vi "Autonomous Independent.vi"   [LabVIEW 2011]
doc: "This VI is called when autonomous begins, and will automatically be terminated when autonomous ends. You can carry out timed or sensor driven robot movement independently without needing to return to the caller."
uses:
  Robot Global Data.vi
  System Set Points and States.vi
types:
  T1 = typedef "WPI_DigitalInputDevRef.ctl" = cluster{"DevStatus":errorcluster, "DIO Channel":T2, "Digital Module":T3}
  T2 = typedef "FPGA_DIOChannel.ctl" = enum8{"DIO 1", "DIO 2", "DIO 3", "DIO 4", "DIO 5", "DIO 6", "DIO 7", "DIO 8", "DIO 9", "DIO 10", "DIO 11", "DIO 12", "DIO 13", "DIO 14", "Invalid"}
  T3 = typedef "FPGA_TypedefDigitalModule.ctl" = enum16{"Digital Module 1", "Digital Module 2"}
  T4 = typedef "WPI_MotorControlDeviceRef.ctl" = cluster{"DeviceStatus":errorcluster, "Type":enum16{"PWM", "CAN"}, "PWM":cluster{"Digital Module":T3, "PWM Channel":T5, "DeadBand":T6}, "CAN":cluster{"Device Number":u8, "Control Mode":T7, "Semaphore":T8, "Max Vout":dbl}, "Invert":bool, "TransformRef":T9, "InvTransformRef":T9}
  T5 = typedef "FPGA_DIOPWMChannel.ctl" = enum8{"PWM 1", "PWM 2", "PWM 3", "PWM 4", "PWM 5", "PWM 6", "PWM 7", "PWM 8", "PWM 9", "PWM 10", "Invalid"}
  T6 = typedef "WPI_PWMDeadband.ctl" = cluster{"Name":string, "maxPositivePwm":i32, "minPositivePwm":i32, "centerPwm":i32, "maxNegativePwm":i32, "minNegativePwm":i32, "angularRange":u16}
  T7 = typedef "WPI_CANJaguar_ControlMode.ctl" = enum8{"Percent VBus", "Current", "Speed", "Position", "Voltage"}
  T8 = typedef "Semaphore RefNum" = refnum<k1>
  T9 = typedef "WPI_PWMTransform_ConPane.ctl" = refnum<vi>
  T10 = typedef "WPI_AnalogChannelDevRef.ctl" = cluster{"DevStatus":errorcluster, "Analog Module":T11, "Analog Channel":T12}
  T11 = typedef "FPGA_TypedefAnalogModule.ctl" = enum16{"Analog Module 1", "Analog Module 2"}
  T12 = typedef "FPGA_AIChannel.ctl" = enum8{"AI 1", "AI 2", "AI 3", "AI 4", "AI 5", "AI 6", "AI 7", "AI 8", "Invalid"}
  T13 = typedef "WPI_RobotDriveDevRef.ctl" = cluster{"DevStatus":errorcluster, "Motors[]":T4[], "Square Inputs":bool, "Max Output":dbl, "Isochronous":bool}
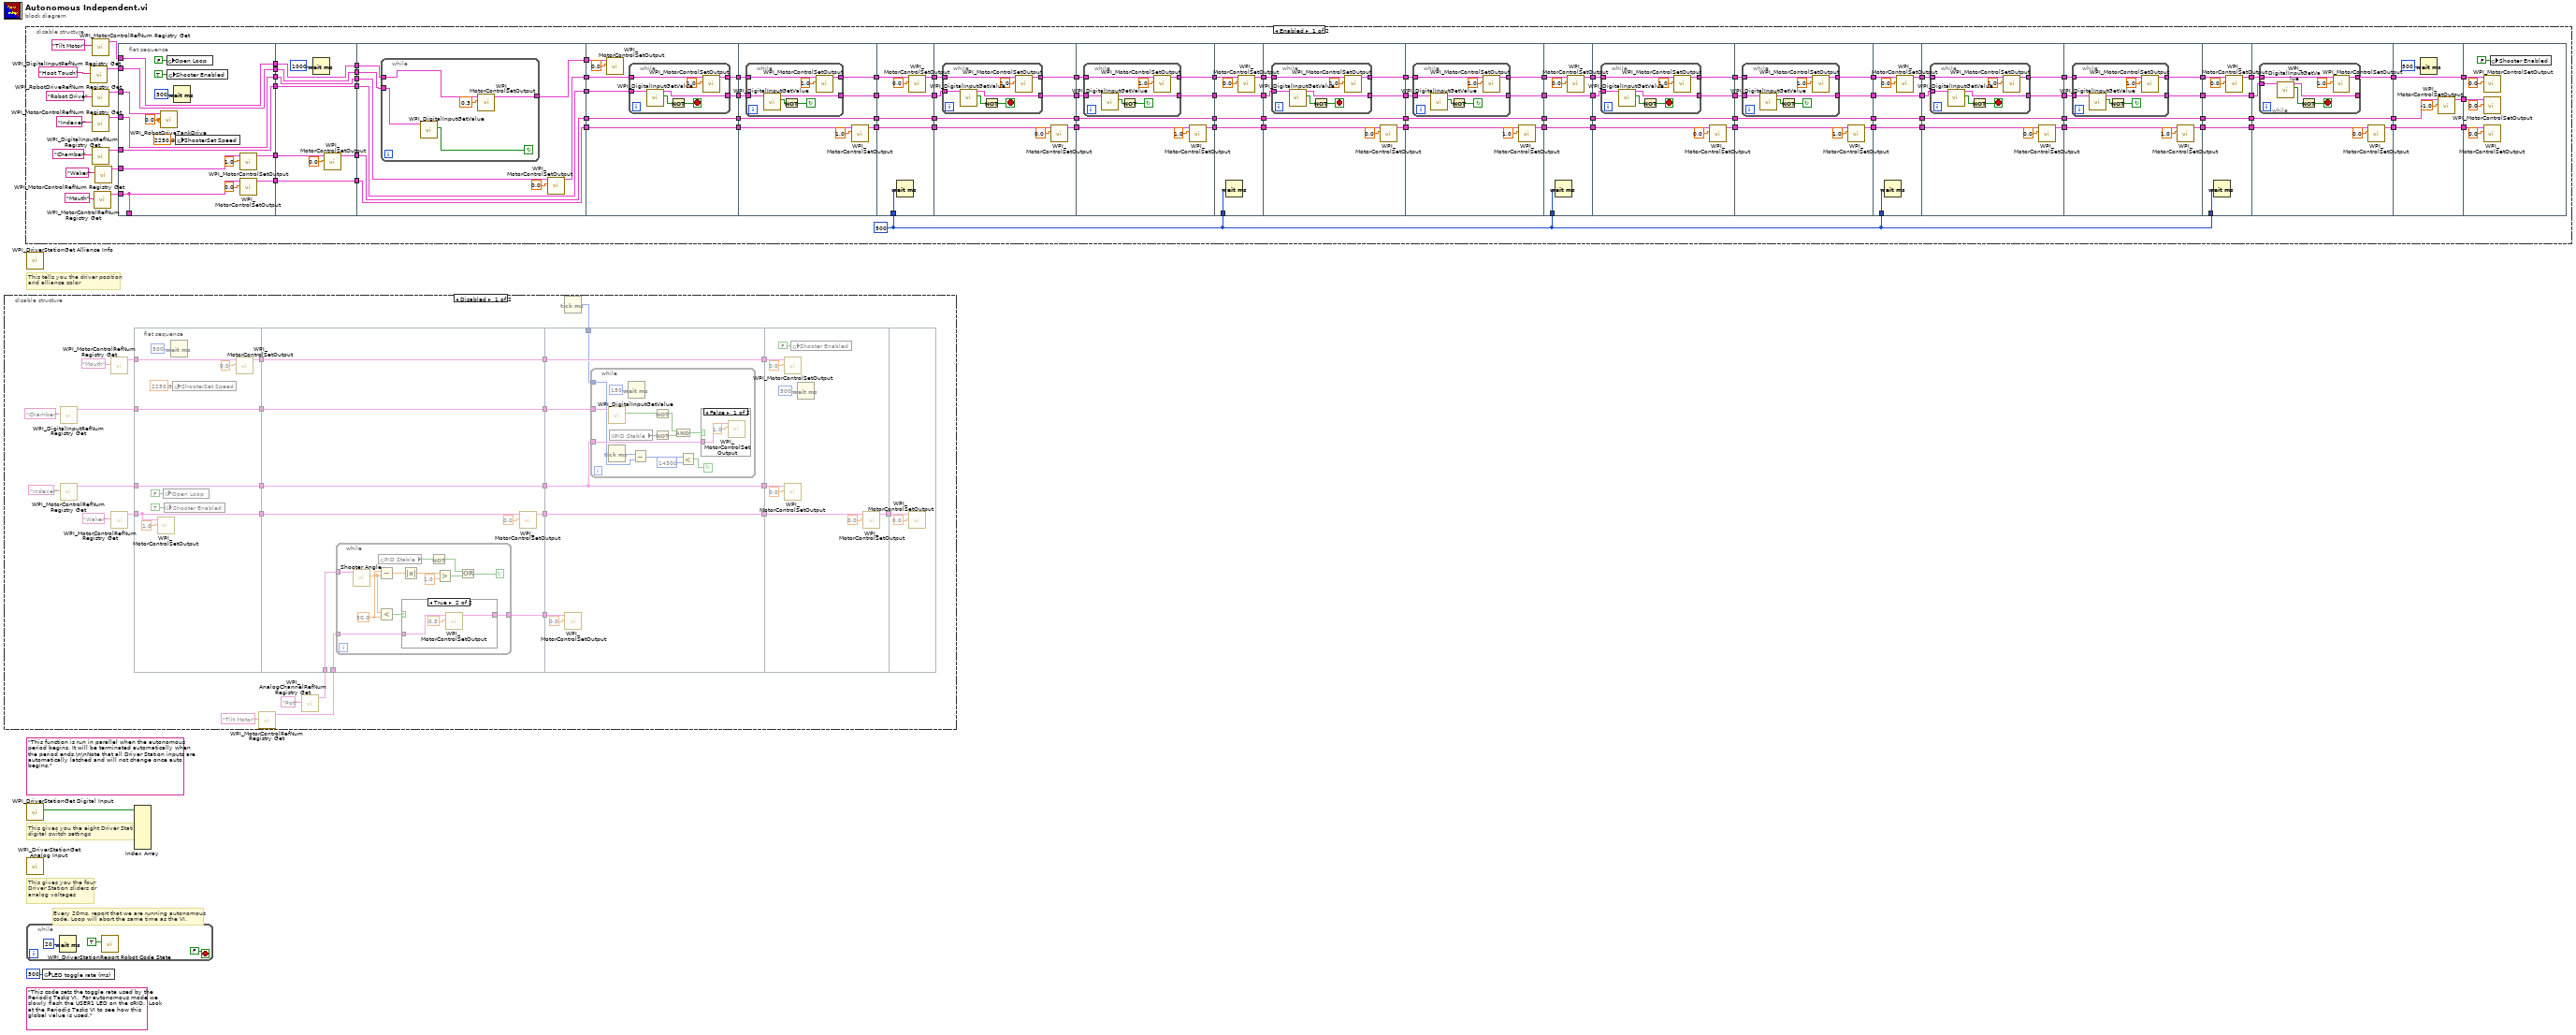
[diagram p0: block diagram]
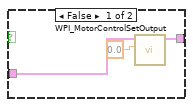
[diagram p2: hidden frame]
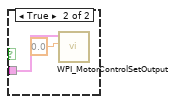
[diagram p3: hidden frame]
diagram:
  (unwired) "This function is run in parallel when the autonomous period begins. It will be terminated automatically when the period ends.\n\nNote that all Driver Station inputs are automatically latched and will not change once auto begins."
  (unwired) "This code sets the toggle rate used by the Periodic Tasks VI.  For autonomous mode we slowly flash the USER1 LED on the cRIO.  Look at the Periodic Tasks VI to see how this global value is used."
  # "Every 20ms, report that we are running autonomous\ncode. Loop will abort the same time as the VI."
  # "This tells you the driver position\nand alliance color"
  # "This gives you the eight Driver Station\ndigital switch settings"
  # "This gives you the four\nDriver Station sliders or\nanalog voltages"
  n1 = disable-structure shown="Disabled" {
    frame Disabled {
      n2 = call <vilib>:"WPI_DigitalInputRefNum Registry Get.vi"("refnum name"="Chamber") -> ("DigitalInputDevRef"=w12:T1)  [unwired: 9 in, 1 out]
      n3 = call <vilib>:"WPI_MotorControlRefNum Registry Get.vi"("refnum name"="Indexer") -> ("MotorControlDevRef"=w9:T4)  [unwired: 9 in, 1 out]
      n4 = call <vilib>:"WPI_MotorControlRefNum Registry Get.vi"("refnum name"="Mouth") -> ("MotorControlDevRef"=w7:T4)  [unwired: 9 in, 1 out]
      n5 = call <vilib>:"WPI_MotorControlRefNum Registry Get.vi"("refnum name"="Waker") -> ("MotorControlDevRef"=w8:T4)  [unwired: 9 in, 1 out]
      n6 = flat-sequence {
        tunnel: w9 -> [w34]
        tunnel: w8 -> [w32]
        tunnel: w12 -> [w33]
        tunnel: [w34] -> w28
        tunnel: [w33] -> w27
        tunnel: [w32] -> w26
        tunnel: w7 -> [w30]
        tunnel: [w29] -> w25
        tunnel: w28 -> [w48]
        tunnel: [w48] -> w24
        tunnel: w27 -> [w47]
        tunnel: [w47] -> w23
        tunnel: w26 -> [w46]
        tunnel: [w44] -> w22
        tunnel: w25 -> [w44]
        tunnel: w5 -> [w43]
        tunnel: w3 -> [w42]
        tunnel: [w41] -> w21
        tunnel: [w40] -> w20
        tunnel: w24 -> [w73]
        tunnel: w23 -> [w74]
        tunnel: [w73] -> w19
        tunnel: [w72] -> w18
        tunnel: w22 -> [w72]
        tunnel: w10 -> [w71]
        tunnel: w21 -> [w69]
        tunnel: [w68] -> w17
        tunnel: w20 -> [w68]
        tunnel: w19 -> [w98]
        tunnel: w18 -> [w96]
        tunnel: w17 -> [w93]
        tunnel: [w92] -> w16
        tunnel: w16 -> [w102]
        frame #0 {
          n7 = call <vilib>:"WPI_MotorControlSetOutput.vi"("Output"=1.0, "MotorControlDevRef"=w32) -> ()  [unwired: 8 in, 2 out]
          n8 = global write "System Set Points and States.vi" "Open Loop"(FALSE ("Open Loop")) -> ()
          n9 = global write "System Set Points and States.vi" "Shooter Enabled"(TRUE ("Shooter Enabled")) -> ()
          n10 = Wait (ms)(milliseconds to wait=u32 500) -> ()  [unwired: 1 out]
          n11 = global write "System Set Points and States.vi" "ShooterSet Speed"(2250.0) -> ()
          n12 = call <vilib>:"WPI_MotorControlSetOutput.vi"("Output"=0.0, "MotorControlDevRef"=w30) -> ("MotorControlDevRef"=w29:T4)  [unwired: 8 in, 1 out]
        }
        frame #1 {
          n13 = while {
            tunnel: w43 -> [w56]
            tunnel: w42 -> [w55]
            tunnel: [w54] -> w41
            stop <- w49 continue-if-true
            w58 = 50.0 ("y")
            n14 = call "Shooter Angle.vi"("AIDeviceRef"=w56) -> ("Shoter Angle"=w57:dbl)  [unwired: 9 in, 1 out]
            n15 = Subtract(x=w58, y=w57) -> (x-y=w59:dbl)
            n16 = Less?(x=w57, y=w58) -> (x < y?=w60:bool)
            n17 = global read "System Set Points and States.vi" "PID Stable"() -> (w61:bool)
            n18 = case shown="True" w60 {
              tunnel: w55 -> [w63 w66]
              tunnel: [w62 w65] -> w54
              frame False {
                n19 = call <vilib>:"WPI_MotorControlSetOutput.vi"("Output"=0.0, "MotorControlDevRef"=w63) -> ("MotorControlDevRef"=w62:T4)  [unwired: 8 in, 1 out]
              }
              frame True {
                n20 = call <vilib>:"WPI_MotorControlSetOutput.vi"("Output"=0.3, "MotorControlDevRef"=w66) -> ("MotorControlDevRef"=w65:T4)  [unwired: 8 in, 1 out]
              }
            }
            n21 = Absolute Value(x=w59) -> (abs(x)=w53:dbl)
            n22 = Not(x=w61) -> (.not. x?=w50:bool)
            n23 = Greater?(x=w53, y=1.0) -> (0:w51:bool)
            n24 = Or(x=w50, y=w51) -> (x .or. y?=w49:bool)
          }
          n25 = call <vilib>:"WPI_MotorControlSetOutput.vi"("Output"=0.0, "MotorControlDevRef"=w46) -> ("MotorControlDevRef"=w40:T4)  [unwired: 8 in, 1 out]
        }
        frame #2 {
          n26 = call <vilib>:"WPI_MotorControlSetOutput.vi"("Output"=0.0, "MotorControlDevRef"=w69) -> ()  [unwired: 8 in, 2 out]
          n27 = while {
            tunnel: w74 -> [w87]
            tunnel: w73 -> [w86]
            tunnel: w71 -> [w77]
            stop <- w84 continue-if-true
            n28 = call <vilib>:"WPI_DigitalInputGetValue.vi"("DigitalInputDevRef"=w87) -> ("Value"=w83:bool)  [unwired: 8 in, 2 out]
            n29 = Tick Count (ms)() -> (millisecond timer value=w76:u32)
            n30 = global read "System Set Points and States.vi" "PID Stable"() -> (w81:bool)
            n31 = Wait (ms)(milliseconds to wait=u32 150) -> ()  [unwired: 1 out]
            n32 = Subtract(x=w76, y=w77) -> (x-y=w78:u32)
            n33 = Not(x=w83) -> (.not. x?=w82:bool)
            n34 = Not(x=w81) -> (.not. x?=w80:bool)
            n35 = And(x=w82, y=w80) -> (x .and. y?=w79:bool)
            n36 = Less?(x=w78, y=u32 14300) -> (x < y?=w84:bool)
            n37 = case shown="False" w79 {
              tunnel: w86 -> [w89 w91]
              frame False {
                n38 = call <vilib>:"WPI_MotorControlSetOutput.vi"("Output"=1.0, "MotorControlDevRef"=w89) -> ()  [unwired: 8 in, 2 out]
              }
              frame True {
                n39 = call <vilib>:"WPI_MotorControlSetOutput.vi"("Output"=0.0, "MotorControlDevRef"=w91) -> ()  [unwired: 8 in, 2 out]
              }
            }
          }
        }
        frame #3 {
          n40 = call <vilib>:"WPI_MotorControlSetOutput.vi"("Output"=0.0, "MotorControlDevRef"=w96) -> ()  [unwired: 8 in, 2 out]
          n41 = call <vilib>:"WPI_MotorControlSetOutput.vi"("Output"=0.0, "MotorControlDevRef"=w98) -> ()  [unwired: 8 in, 2 out]
          n42 = global write "System Set Points and States.vi" "Shooter Enabled"(FALSE ("Shooter Enabled")) -> ()
          n43 = Wait (ms)(milliseconds to wait=u32 500) -> ()  [unwired: 1 out]
          n44 = call <vilib>:"WPI_MotorControlSetOutput.vi"("Output"=0.0, "MotorControlDevRef"=w93) -> ("MotorControlDevRef"=w92:T4)  [unwired: 8 in, 1 out]
        }
        frame #4 {
          n45 = call <vilib>:"WPI_MotorControlSetOutput.vi"("Output"=0.0, "MotorControlDevRef"=w102) -> ()  [unwired: 8 in, 2 out]
        }
      }
      n46 = call <vilib>:"WPI_MotorControlRefNum Registry Get.vi"("refnum name"="Tilt Motor") -> ("MotorControlDevRef"=w3:T4)  [unwired: 9 in, 1 out]
      n47 = call <vilib>:"WPI_AnalogChannelRefNum Registry Get.vi"("refnum name"="Pot") -> ("AIDeviceRef"=w5:T10)  [unwired: 9 in, 1 out]
      n48 = Tick Count (ms)() -> (millisecond timer value=w10:u32)
    }
    frame Enabled {
    }
  }
  n49 = disable-structure shown="Enabled" {
    frame Enabled {
      w107 = u32 500 ("milliseconds to wait")
      n50 = call <vilib>:"WPI_DigitalInputRefNum Registry Get.vi"("refnum name"="Hoot Touch") -> ("DigitalInputDevRef"=w103:T1)  [unwired: 9 in, 1 out]
      n51 = call <vilib>:"WPI_MotorControlRefNum Registry Get.vi"("refnum name"="Tilt Motor") -> ("MotorControlDevRef"=w113:T4)  [unwired: 9 in, 1 out]
      n52 = call <vilib>:"WPI_RobotDriveRefNum Registry Get.vi"("refnum name"="Robot Drive") -> ("RobotDriveDevRef"=w108:T13)  [unwired: 9 in, 1 out]
      n53 = call <vilib>:"WPI_MotorControlRefNum Registry Get.vi"("refnum name"="Indexer") -> ("MotorControlDevRef"=w112:T4)  [unwired: 9 in, 1 out]
      n54 = call <vilib>:"WPI_DigitalInputRefNum Registry Get.vi"("refnum name"="Chamber") -> ("DigitalInputDevRef"=w116:T1)  [unwired: 9 in, 1 out]
      n55 = call <vilib>:"WPI_MotorControlRefNum Registry Get.vi"("refnum name"="Mouth") -> ("MotorControlDevRef"=w110:T4)  [unwired: 9 in, 1 out]
      n56 = call <vilib>:"WPI_MotorControlRefNum Registry Get.vi"("refnum name"="Waker") -> ("MotorControlDevRef"=w111:T4)  [unwired: 9 in, 1 out]
      n57 = flat-sequence {
        tunnel: w112 -> [w211]
        tunnel: w111 -> [w209]
        tunnel: w116 -> [w210]
        tunnel: [w211] -> w200
        tunnel: [w210] -> w199
        tunnel: [w202] -> w198
        tunnel: [w205] -> _
        tunnel: [w207] -> w197
        tunnel: [w206] -> w196
        tunnel: w113 -> [w206]
        tunnel: w110 -> [w205]
        tunnel: w108 -> [w204]
        tunnel: [w201] -> w104
        tunnel: w103 -> [w201]
        tunnel: w200 -> [w225]
        tunnel: [w225] -> w195
        tunnel: w199 -> [w224]
        tunnel: [w224] -> w194
        tunnel: w198 -> [w220]
        tunnel: w197 -> [w223]
        tunnel: [w223] -> w193
        tunnel: w196 -> [w222]
        tunnel: [w222] -> w192
        tunnel: [w219] -> w191
        tunnel: [w217] -> w105
        tunnel: w104 -> [w217]
        tunnel: w195 -> [w230]
        tunnel: [w228] -> w190
        tunnel: w194 -> [w234]
        tunnel: [w234] -> w189
        tunnel: [w233] -> w188
        tunnel: w193 -> [w233]
        tunnel: w192 -> [w232]
        tunnel: [w231] -> w187
        tunnel: [w227] -> w186
        tunnel: w191 -> [w227]
        tunnel: w105 -> [w226]
        tunnel: w190 -> [w247]
        tunnel: w189 -> [w242]
        tunnel: [w244] -> w185
        tunnel: [w243] -> w184
        tunnel: w188 -> [w243]
        tunnel: w187 -> [w245]
        tunnel: [w241] -> w183
        tunnel: [w240] -> w182
        tunnel: w186 -> [w240]
        tunnel: w185 -> [w262]
        tunnel: w184 -> [w257]
        tunnel: w183 -> [w261]
        tunnel: [w260] -> w181
        tunnel: [w259] -> w180
        tunnel: [w256] -> w179
        tunnel: [w255] -> w178
        tunnel: w182 -> [w255]
        tunnel: [w271] -> w177
        tunnel: w181 -> [w273]
        tunnel: w180 -> [w275]
        tunnel: w179 -> [w271]
        tunnel: [w274] -> w176
        tunnel: [w273] -> w175
        tunnel: w107 -> [w272]
        tunnel: [w270] -> w174
        tunnel: w178 -> [w270]
        tunnel: w177 -> [w279]
        tunnel: [w278] -> w173
        tunnel: w176 -> [w284]
        tunnel: [w283] -> w172
        tunnel: [w282] -> w171
        tunnel: w175 -> [w281]
        tunnel: [w277] -> w170
        tunnel: w174 -> [w277]
        tunnel: w173 -> [w298]
        tunnel: w172 -> [w297]
        tunnel: w171 -> [w296]
        tunnel: [w295] -> w169
        tunnel: [w294] -> w168
        tunnel: [w293] -> w167
        tunnel: [w292] -> w166
        tunnel: w170 -> [w292]
        tunnel: w169 -> [w312]
        tunnel: [w311] -> w165
        tunnel: w168 -> [w311]
        tunnel: [w310] -> w164
        tunnel: w167 -> [w308]
        tunnel: [w308] -> w163
        tunnel: w107 -> [w309]
        tunnel: [w307] -> w162
        tunnel: w166 -> [w307]
        tunnel: w165 -> [w320]
        tunnel: w164 -> [w321]
        tunnel: w163 -> [w316]
        tunnel: [w315] -> w161
        tunnel: [w319] -> w160
        tunnel: [w318] -> w159
        tunnel: [w314] -> w158
        tunnel: w162 -> [w314]
        tunnel: w161 -> [w331]
        tunnel: w160 -> [w336]
        tunnel: w159 -> [w335]
        tunnel: [w330] -> w157
        tunnel: [w334] -> w156
        tunnel: [w333] -> w155
        tunnel: [w329] -> w154
        tunnel: w158 -> [w329]
        tunnel: w157 -> [w345]
        tunnel: w156 -> [w347]
        tunnel: w155 -> [w349]
        tunnel: w107 -> [w348]
        tunnel: [w347] -> w153
        tunnel: [w346] -> w152
        tunnel: [w345] -> w151
        tunnel: [w344] -> w150
        tunnel: w154 -> [w344]
        tunnel: w153 -> [w358]
        tunnel: w152 -> [w357]
        tunnel: [w352] -> w149
        tunnel: w151 -> [w353]
        tunnel: [w356] -> w148
        tunnel: [w355] -> w147
        tunnel: [w351] -> w146
        tunnel: w150 -> [w351]
        tunnel: w149 -> [w368]
        tunnel: [w367] -> w145
        tunnel: w148 -> [w373]
        tunnel: w147 -> [w372]
        tunnel: [w371] -> w144
        tunnel: [w370] -> w143
        tunnel: [w366] -> w142
        tunnel: w146 -> [w366]
        tunnel: w145 -> [w382]
        tunnel: [w382] -> w141
        tunnel: [w385] -> w140
        tunnel: w144 -> [w386]
        tunnel: w107 -> [w384]
        tunnel: w143 -> [w383]
        tunnel: [w383] -> w139
        tunnel: [w381] -> w138
        tunnel: w142 -> [w381]
        tunnel: w141 -> [w390]
        tunnel: [w389] -> w137
        tunnel: w140 -> [w395]
        tunnel: [w393] -> w136
        tunnel: w139 -> [w394]
        tunnel: [w392] -> w135
        tunnel: [w388] -> w134
        tunnel: w138 -> [w388]
        tunnel: w137 -> [w405]
        tunnel: [w404] -> w133
        tunnel: w136 -> [w410]
        tunnel: [w408] -> w132
        tunnel: w135 -> [w409]
        tunnel: [w407] -> w131
        tunnel: [w403] -> w130
        tunnel: w134 -> [w403]
        tunnel: w133 -> [w419]
        tunnel: [w419] -> w129
        tunnel: w132 -> [w422]
        tunnel: [w423] -> w128
        tunnel: w107 -> [w421]
        tunnel: w131 -> [w420]
        tunnel: [w420] -> w127
        tunnel: [w418] -> w126
        tunnel: w130 -> [w418]
        tunnel: w129 -> [w427]
        tunnel: [w426] -> w125
        tunnel: w128 -> [w430]
        tunnel: [w431] -> w124
        tunnel: w127 -> [w429]
        tunnel: [w425] -> w123
        tunnel: w126 -> [w425]
        tunnel: w125 -> [w444]
        tunnel: [w444] -> w122
        tunnel: w124 -> [w443]
        tunnel: [w443] -> w121
        tunnel: w123 -> [w442]
        tunnel: [w440] -> w120
        tunnel: w122 -> [w449]
        tunnel: w121 -> [w447]
        tunnel: w120 -> [w446]
        frame #0 {
          w203 = 0.0 ("Left axis value")
          n58 = call <vilib>:"WPI_RobotDriveTankDrive.vi"("Right axis value"=w203, "Left axis value"=w203, "RobotDriveDevRef"=w204) -> ()  [unwired: 7 in, 2 out]
          n59 = global write "System Set Points and States.vi" "Open Loop"(FALSE ("Open Loop")) -> ()
          n60 = global write "System Set Points and States.vi" "Shooter Enabled"(TRUE ("Shooter Enabled")) -> ()
          n61 = Wait (ms)(milliseconds to wait=u32 500) -> ()  [unwired: 1 out]
          n62 = global write "System Set Points and States.vi" "ShooterSet Speed"(2250.0) -> ()
          n63 = call <vilib>:"WPI_MotorControlSetOutput.vi"("Output"=1.0, "MotorControlDevRef"=w209) -> ("MotorControlDevRef"=w202:T4)  [unwired: 8 in, 1 out]
          n64 = call <vilib>:"WPI_MotorControlSetOutput.vi"("Output"=0.0, "MotorControlDevRef"=w205) -> ("MotorControlDevRef"=w207:T4)  [unwired: 8 in, 1 out]
        }
        frame #1 {
          n65 = Wait (ms)(milliseconds to wait=u32 1000) -> ()  [unwired: 1 out]
          n66 = call <vilib>:"WPI_MotorControlSetOutput.vi"("Output"=0.0, "MotorControlDevRef"=w220) -> ("MotorControlDevRef"=w219:T4)  [unwired: 8 in, 1 out]
        }
        frame #2 {
          n67 = while {
            tunnel: w232 -> [w239]
            tunnel: [w238] -> w231
            tunnel: w226 -> [w236]
            stop <- w235 continue-if-true
            n68 = call <vilib>:"WPI_DigitalInputGetValue.vi"("DigitalInputDevRef"=w236) -> ("Value"=w235:bool)  [unwired: 8 in, 2 out]
            n69 = call <vilib>:"WPI_MotorControlSetOutput.vi"("Output"=0.3, "MotorControlDevRef"=w239) -> ("MotorControlDevRef"=w238:T4)  [unwired: 8 in, 1 out]
          }
          n70 = call <vilib>:"WPI_MotorControlSetOutput.vi"("Output"=0.0, "MotorControlDevRef"=w230) -> ("MotorControlDevRef"=w228:T4)  [unwired: 8 in, 1 out]
        }
        frame #3 {
          n71 = call <vilib>:"WPI_MotorControlSetOutput.vi"("Output"=0.0, "MotorControlDevRef"=w245) -> ()  [unwired: 8 in, 2 out]
          n72 = while {
            tunnel: w247 -> [w254]
            tunnel: [w253] -> w244
            tunnel: w242 -> [w250]
            tunnel: [w248] -> w241
            stop <- w249 stop-if-true
            n73 = call <vilib>:"WPI_DigitalInputGetValue.vi"("DigitalInputDevRef"=w250) -> ("Value"=w251:bool, "DigitalInputDevRef"=w248:T1)  [unwired: 8 in, 1 out]
            n74 = Not(x=w251) -> (.not. x?=w249:bool)
            n75 = call <vilib>:"WPI_MotorControlSetOutput.vi"("Output"=1.0, "MotorControlDevRef"=w254) -> ("MotorControlDevRef"=w253:T4)  [unwired: 8 in, 1 out]
          }
        }
        frame #4 {
          n76 = while {
            tunnel: w262 -> [w269]
            tunnel: [w268] -> w259
            tunnel: w261 -> [w265]
            tunnel: [w263] -> w260
            stop <- w264 continue-if-true
            n77 = call <vilib>:"WPI_DigitalInputGetValue.vi"("DigitalInputDevRef"=w265) -> ("Value"=w266:bool, "DigitalInputDevRef"=w263:T1)  [unwired: 8 in, 1 out]
            n78 = Not(x=w266) -> (.not. x?=w264:bool)
            n79 = call <vilib>:"WPI_MotorControlSetOutput.vi"("Output"=1.0, "MotorControlDevRef"=w269) -> ("MotorControlDevRef"=w268:T4)  [unwired: 8 in, 1 out]
          }
          n80 = call <vilib>:"WPI_MotorControlSetOutput.vi"("Output"=1.0, "MotorControlDevRef"=w257) -> ("MotorControlDevRef"=w256:T4)  [unwired: 8 in, 1 out]
        }
        frame #5 {
          n81 = Wait (ms)(milliseconds to wait=w272) -> ()  [unwired: 1 out]
          n82 = call <vilib>:"WPI_MotorControlSetOutput.vi"("Output"=0.0, "MotorControlDevRef"=w275) -> ("MotorControlDevRef"=w274:T4)  [unwired: 8 in, 1 out]
        }
        frame #6 {
          n83 = while {
            tunnel: [w291] -> w282
            tunnel: [w287] -> w283
            tunnel: w284 -> [w286]
            tunnel: w281 -> [w285]
            stop <- w288 stop-if-true
            n84 = call <vilib>:"WPI_DigitalInputGetValue.vi"("DigitalInputDevRef"=w285) -> ("Value"=w289:bool, "DigitalInputDevRef"=w287:T1)  [unwired: 8 in, 1 out]
            n85 = Not(x=w289) -> (.not. x?=w288:bool)
            n86 = call <vilib>:"WPI_MotorControlSetOutput.vi"("Output"=1.0, "MotorControlDevRef"=w286) -> ("MotorControlDevRef"=w291:T4)  [unwired: 8 in, 1 out]
          }
          n87 = call <vilib>:"WPI_MotorControlSetOutput.vi"("Output"=0.0, "MotorControlDevRef"=w279) -> ("MotorControlDevRef"=w278:T4)  [unwired: 8 in, 1 out]
        }
        frame #7 {
          n88 = while {
            tunnel: [w306] -> w295
            tunnel: [w302] -> w294
            tunnel: w296 -> [w301]
            tunnel: w297 -> [w300]
            stop <- w303 continue-if-true
            n89 = call <vilib>:"WPI_DigitalInputGetValue.vi"("DigitalInputDevRef"=w300) -> ("Value"=w304:bool, "DigitalInputDevRef"=w302:T1)  [unwired: 8 in, 1 out]
            n90 = Not(x=w304) -> (.not. x?=w303:bool)
            n91 = call <vilib>:"WPI_MotorControlSetOutput.vi"("Output"=1.0, "MotorControlDevRef"=w301) -> ("MotorControlDevRef"=w306:T4)  [unwired: 8 in, 1 out]
          }
          n92 = call <vilib>:"WPI_MotorControlSetOutput.vi"("Output"=1.0, "MotorControlDevRef"=w298) -> ("MotorControlDevRef"=w293:T4)  [unwired: 8 in, 1 out]
        }
        frame #8 {
          n93 = Wait (ms)(milliseconds to wait=w309) -> ()  [unwired: 1 out]
          n94 = call <vilib>:"WPI_MotorControlSetOutput.vi"("Output"=0.0, "MotorControlDevRef"=w312) -> ("MotorControlDevRef"=w310:T4)  [unwired: 8 in, 1 out]
        }
        frame #9 {
          n95 = while {
            tunnel: [w328] -> w318
            tunnel: [w324] -> w319
            tunnel: w321 -> [w323]
            tunnel: w320 -> [w322]
            stop <- w325 stop-if-true
            n96 = call <vilib>:"WPI_DigitalInputGetValue.vi"("DigitalInputDevRef"=w322) -> ("Value"=w326:bool, "DigitalInputDevRef"=w324:T1)  [unwired: 8 in, 1 out]
            n97 = Not(x=w326) -> (.not. x?=w325:bool)
            n98 = call <vilib>:"WPI_MotorControlSetOutput.vi"("Output"=1.0, "MotorControlDevRef"=w323) -> ("MotorControlDevRef"=w328:T4)  [unwired: 8 in, 1 out]
          }
          n99 = call <vilib>:"WPI_MotorControlSetOutput.vi"("Output"=0.0, "MotorControlDevRef"=w316) -> ("MotorControlDevRef"=w315:T4)  [unwired: 8 in, 1 out]
        }
        frame #10 {
          n100 = while {
            tunnel: [w343] -> w333
            tunnel: [w339] -> w334
            tunnel: w335 -> [w338]
            tunnel: w336 -> [w337]
            stop <- w340 continue-if-true
            n101 = call <vilib>:"WPI_DigitalInputGetValue.vi"("DigitalInputDevRef"=w337) -> ("Value"=w341:bool, "DigitalInputDevRef"=w339:T1)  [unwired: 8 in, 1 out]
            n102 = Not(x=w341) -> (.not. x?=w340:bool)
            n103 = call <vilib>:"WPI_MotorControlSetOutput.vi"("Output"=1.0, "MotorControlDevRef"=w338) -> ("MotorControlDevRef"=w343:T4)  [unwired: 8 in, 1 out]
          }
          n104 = call <vilib>:"WPI_MotorControlSetOutput.vi"("Output"=1.0, "MotorControlDevRef"=w331) -> ("MotorControlDevRef"=w330:T4)  [unwired: 8 in, 1 out]
        }
        frame #11 {
          n105 = Wait (ms)(milliseconds to wait=w348) -> ()  [unwired: 1 out]
          n106 = call <vilib>:"WPI_MotorControlSetOutput.vi"("Output"=0.0, "MotorControlDevRef"=w349) -> ("MotorControlDevRef"=w346:T4)  [unwired: 8 in, 1 out]
        }
        frame #12 {
          n107 = while {
            tunnel: [w365] -> w356
            tunnel: [w361] -> w355
            tunnel: w357 -> [w360]
            tunnel: w358 -> [w359]
            stop <- w362 stop-if-true
            n108 = call <vilib>:"WPI_DigitalInputGetValue.vi"("DigitalInputDevRef"=w359) -> ("Value"=w363:bool, "DigitalInputDevRef"=w361:T1)  [unwired: 8 in, 1 out]
            n109 = Not(x=w363) -> (.not. x?=w362:bool)
            n110 = call <vilib>:"WPI_MotorControlSetOutput.vi"("Output"=1.0, "MotorControlDevRef"=w360) -> ("MotorControlDevRef"=w365:T4)  [unwired: 8 in, 1 out]
          }
          n111 = call <vilib>:"WPI_MotorControlSetOutput.vi"("Output"=0.0, "MotorControlDevRef"=w353) -> ("MotorControlDevRef"=w352:T4)  [unwired: 8 in, 1 out]
        }
        frame #13 {
          n112 = while {
            tunnel: [w380] -> w371
            tunnel: [w376] -> w370
            tunnel: w373 -> [w375]
            tunnel: w372 -> [w374]
            stop <- w377 continue-if-true
            n113 = call <vilib>:"WPI_DigitalInputGetValue.vi"("DigitalInputDevRef"=w374) -> ("Value"=w378:bool, "DigitalInputDevRef"=w376:T1)  [unwired: 8 in, 1 out]
            n114 = Not(x=w378) -> (.not. x?=w377:bool)
            n115 = call <vilib>:"WPI_MotorControlSetOutput.vi"("Output"=1.0, "MotorControlDevRef"=w375) -> ("MotorControlDevRef"=w380:T4)  [unwired: 8 in, 1 out]
          }
          n116 = call <vilib>:"WPI_MotorControlSetOutput.vi"("Output"=1.0, "MotorControlDevRef"=w368) -> ("MotorControlDevRef"=w367:T4)  [unwired: 8 in, 1 out]
        }
        frame #14 {
          n117 = Wait (ms)(milliseconds to wait=w384) -> ()  [unwired: 1 out]
          n118 = call <vilib>:"WPI_MotorControlSetOutput.vi"("Output"=0.0, "MotorControlDevRef"=w386) -> ("MotorControlDevRef"=w385:T4)  [unwired: 8 in, 1 out]
        }
        frame #15 {
          n119 = while {
            tunnel: [w402] -> w393
            tunnel: [w398] -> w392
            tunnel: w395 -> [w397]
            tunnel: w394 -> [w396]
            stop <- w399 stop-if-true
            n120 = call <vilib>:"WPI_DigitalInputGetValue.vi"("DigitalInputDevRef"=w396) -> ("Value"=w400:bool, "DigitalInputDevRef"=w398:T1)  [unwired: 8 in, 1 out]
            n121 = Not(x=w400) -> (.not. x?=w399:bool)
            n122 = call <vilib>:"WPI_MotorControlSetOutput.vi"("Output"=1.0, "MotorControlDevRef"=w397) -> ("MotorControlDevRef"=w402:T4)  [unwired: 8 in, 1 out]
          }
          n123 = call <vilib>:"WPI_MotorControlSetOutput.vi"("Output"=0.0, "MotorControlDevRef"=w390) -> ("MotorControlDevRef"=w389:T4)  [unwired: 8 in, 1 out]
        }
        frame #16 {
          n124 = while {
            tunnel: [w417] -> w408
            tunnel: [w413] -> w407
            tunnel: w409 -> [w412]
            tunnel: w410 -> [w411]
            stop <- w414 continue-if-true
            n125 = call <vilib>:"WPI_DigitalInputGetValue.vi"("DigitalInputDevRef"=w412) -> ("Value"=w415:bool, "DigitalInputDevRef"=w413:T1)  [unwired: 8 in, 1 out]
            n126 = Not(x=w415) -> (.not. x?=w414:bool)
            n127 = call <vilib>:"WPI_MotorControlSetOutput.vi"("Output"=1.0, "MotorControlDevRef"=w411) -> ("MotorControlDevRef"=w417:T4)  [unwired: 8 in, 1 out]
          }
          n128 = call <vilib>:"WPI_MotorControlSetOutput.vi"("Output"=1.0, "MotorControlDevRef"=w405) -> ("MotorControlDevRef"=w404:T4)  [unwired: 8 in, 1 out]
        }
        frame #17 {
          n129 = Wait (ms)(milliseconds to wait=w421) -> ()  [unwired: 1 out]
          n130 = call <vilib>:"WPI_MotorControlSetOutput.vi"("Output"=0.0, "MotorControlDevRef"=w422) -> ("MotorControlDevRef"=w423:T4)  [unwired: 8 in, 1 out]
        }
        frame #18 {
          n131 = while {
            tunnel: [w438] -> w431
            tunnel: [w434] -> _
            tunnel: w430 -> [w433]
            tunnel: w429 -> [w432]
            stop <- w435 stop-if-true
            n132 = call <vilib>:"WPI_DigitalInputGetValue.vi"("DigitalInputDevRef"=w432) -> ("Value"=w436:bool, "DigitalInputDevRef"=w434:T1)  [unwired: 8 in, 1 out]
            n133 = Not(x=w436) -> (.not. x?=w435:bool)
            n134 = call <vilib>:"WPI_MotorControlSetOutput.vi"("Output"=1.0, "MotorControlDevRef"=w433) -> ("MotorControlDevRef"=w438:T4)  [unwired: 8 in, 1 out]
          }
          n135 = call <vilib>:"WPI_MotorControlSetOutput.vi"("Output"=0.0, "MotorControlDevRef"=w427) -> ("MotorControlDevRef"=w426:T4)  [unwired: 8 in, 1 out]
        }
        frame #19 {
          n136 = Wait (ms)(milliseconds to wait=u32 500) -> ()  [unwired: 1 out]
          n137 = call <vilib>:"WPI_MotorControlSetOutput.vi"("Output"=-1.0, "MotorControlDevRef"=w442) -> ("MotorControlDevRef"=w440:T4)  [unwired: 8 in, 1 out]
        }
        frame #20 {
          n138 = call <vilib>:"WPI_MotorControlSetOutput.vi"("Output"=0.0, "MotorControlDevRef"=w447) -> ()  [unwired: 8 in, 2 out]
          n139 = call <vilib>:"WPI_MotorControlSetOutput.vi"("Output"=0.0, "MotorControlDevRef"=w446) -> ()  [unwired: 8 in, 2 out]
          n140 = call <vilib>:"WPI_MotorControlSetOutput.vi"("Output"=0.0, "MotorControlDevRef"=w449) -> ()  [unwired: 8 in, 2 out]
          n141 = global write "System Set Points and States.vi" "Shooter Enabled"(FALSE ("Shooter Enabled")) -> ()
        }
      }
    }
    frame Disabled {
    }
  }
  n142 = call <vilib>:"WPI_DriverStationGet Alliance Info.vi"() -> ()  [unwired: 12 out]
  n143 = call <vilib>:"WPI_DriverStationGet Digital Input.vi"() -> ("Driver Station Digital Input (1-8)"=w2:bool[])  [unwired: 11 out]
  n144 = call <vilib>:"WPI_DriverStationGet Analog Input.vi"() -> ()  [unwired: 12 out]
  n145 = while {
    stop <- FALSE stop-if-true
    n146 = Wait (ms)(milliseconds to wait=u32 20) -> ()  [unwired: 1 out]
    n147 = call <vilib>:"WPI_DriverStationReport Robot Code State.vi"("Autonomous"=TRUE) -> ()  [unwired: 10 in, 1 out]
  }
  n148 = global write "Robot Global Data.vi" "LED toggle rate (ms)"(u32 500 ("LED ms toggle rate")) -> ()
  n149 = Index Array(array=w2) -> ()  [unwired: 8 in, 8 out]
